vi "ALTS-2015 Check Robot Requests.vi"(8 "error in (no error)":errorcluster, 10 "Data Cluster in":T1, 11 "Cases to go in":string) -> (0 "error out":errorcluster, 2 "Data Cluster out":T1, 3 "Cases to go out":string)   [LabVIEW 2013]
uses:
  Controls/ALTS-2015 Data Cluster.ctl
  Controls/ALTS-2015 Station Cluster.ctl
  Controls/ALTS-2015 INI Configuration Cluster.ctl
  Controls/ALTS-2015 Unload Task Data.ctl
  OPC Engine/Controls/ALTS-2015 OPC Read Registers.ctl
  OPC Engine/Controls/ALTS-2015 OPC Read Global Options.ctl
  Controls/ALTS-2015 Auto Main Screen States.ctl
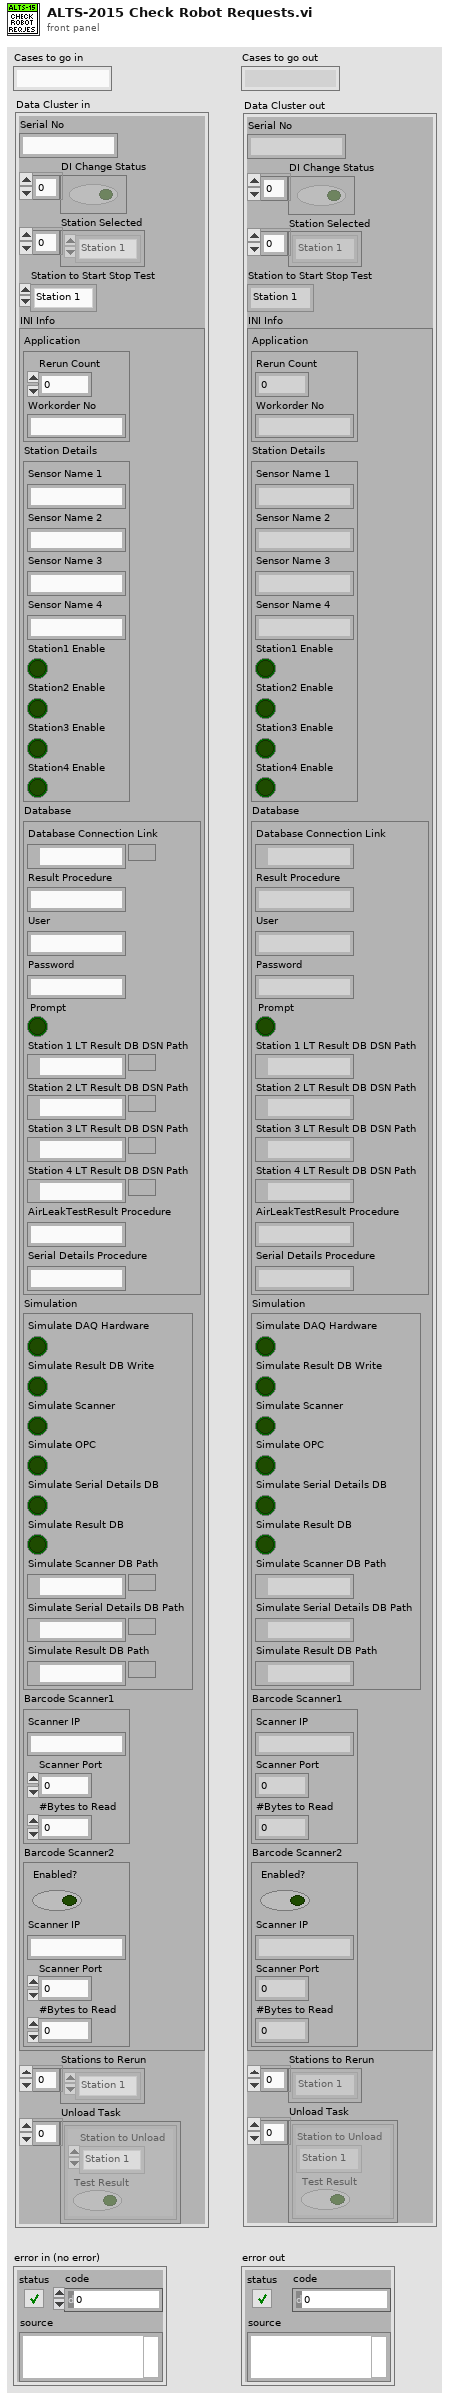
[diagram p1: front panel]
types:
  T1 = typedef "ALTS-2015 Data Cluster.ctl" = cluster{"Serial No":string, "DI Change Status":bool[], "Station Selected":T2[], "Station to Start Stop Test":T2, "INI Info":T3, "Stations to Rerun":T2[], "Unload Task":T4[]}
  T2 = typedef "ALTS-2015 Station Cluster.ctl" = enum16{"Station 1", "Station 2", "Station 3", "Station 4"}
  T3 = typedef "ALTS-2015 INI Configuration Cluster.ctl" = cluster{"Application":cluster{"Rerun Count":i32, "Workorder No":string}, "Station Details":cluster{"Sensor Name 1":string, "Sensor Name 2":string, "Sensor Name 3":string, "Sensor Name 4":string, "Station1 Enable":bool, "Station2 Enable":bool, "Station3 Enable":bool, "Station4 Enable":bool}, "Database":cluster{"Database Connection Link":path, "Result Procedure":string, "User":string, "Password":string, "Prompt":bool, "Station 1 LT Result DB DSN Path":path, "Station 2 LT Result DB DSN Path":path, "Station 3 LT Result DB DSN Path":path, "Station 4 LT Result DB DSN Path":path, "AirLeakTestResult Procedure":string, "Serial Details Procedure":string}, "Simulation":cluster{"Simulate DAQ Hardware":bool, "Simulate Result DB Write":bool, "Simulate Scanner":bool, "Simulate OPC":bool, "Simulate Serial Details DB":bool, "Simulate Result DB":bool, "Simulate Scanner DB Path":path, "Simulate Serial Details DB Path":path, "Simulate Result DB Path":path}, "Barcode Scanner1":cluster{"Scanner IP":string, "Scanner Port":u16, "#Bytes to Read":i32}, "Barcode Scanner2":cluster{"Enabled?":bool, "Scanner IP":string, "Scanner Port":u16, "#Bytes to Read":i32}}
  T4 = typedef "ALTS-2015 Unload Task Data.ctl" = cluster{"Station to Unload":T2, "Test Result":bool}
  T5 = typedef "ALTS-2015 OPC Read Global Options.ctl" = enum16{"Init", "Write Value", "Write Array", "Read Value", "Read Array", "Read All"}
  T6 = typedef "ALTS-2015 OPC Read Registers.ctl" = enum16{"Robot_Available", "Start_Test", "Stop_Test", "Scan_Trigger", "Station_No_Start_Stop_Test"}
  T7 = typedef "ALTS-2015 Auto Main Screen States.ctl" = enum16{">Initialize", ">Poll", ">Error", ">Exit", ">Authentication", ">Initial FP Update", ">Check Robot Requests", ">Scan Serial No", "<-------DI /OPC Actions------->", ">Check DI Status", ">Start the Test", ">Restore station after Stop", ">Stop the Test", ">UUT Clamped", ">UUT Unclamped", ">Read Test Data Result - Pass", ">Read Test Data Result - Fail", ">Update Rerun on Fail", ">Update Station Info", "<--------Enqueue Robot Task-------->", ">Enqueue New Serial Task", ">Enqueue Invalid Serial Task", ">Enqueue Rerun Task", ">Enqueu Unload Task"}
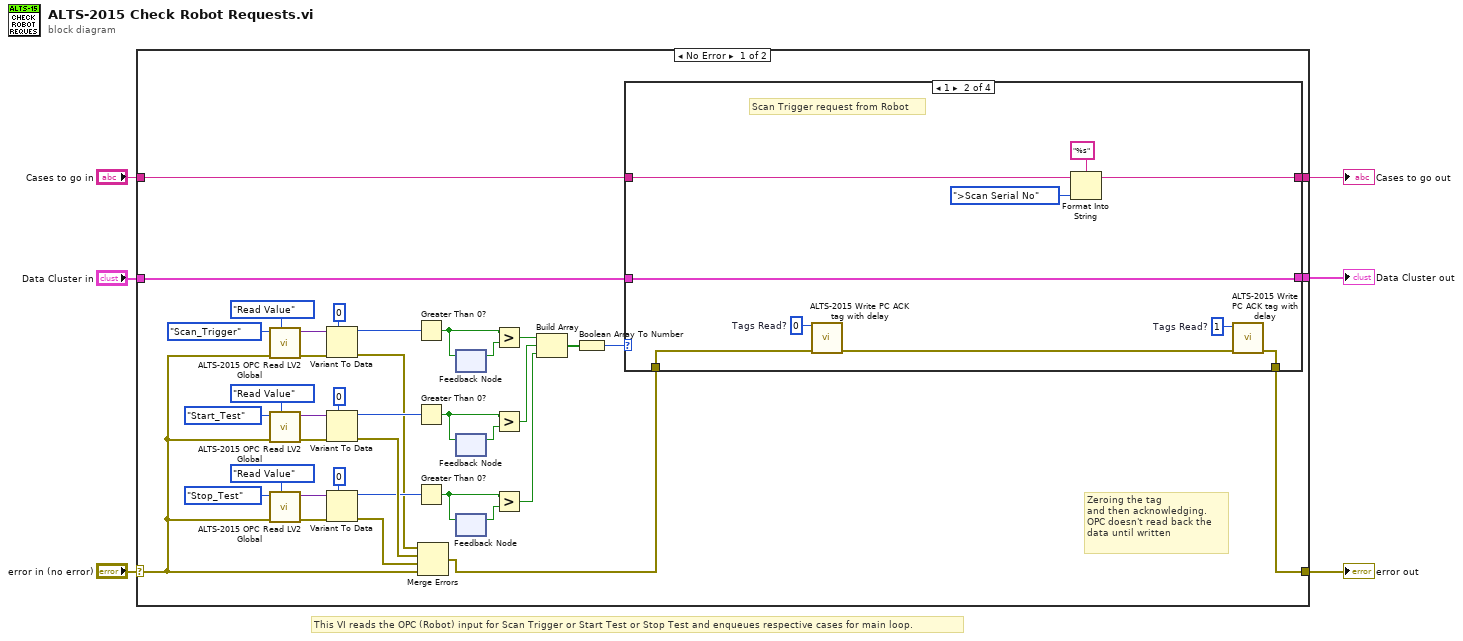
[diagram p0: block diagram]
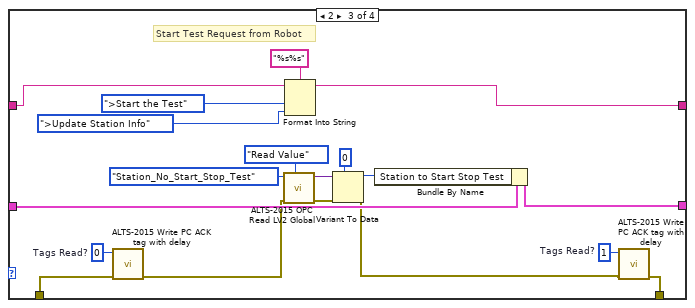
[diagram p3: hidden frame]
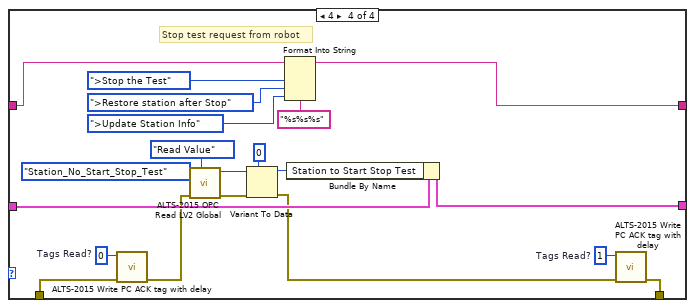
[diagram p4: hidden frame]
diagram:
  # "This VI reads the OPC (Robot) input for Scan Trigger or Start Test or Stop Test and enqueues respective cases for main loop."
  n1 = case shown="No Error" "error in (no error)" {
    selector: "error in (no error)" -> [w11 w100]
    tunnel: [w8 w100] -> w6
    tunnel: [w43 w98] -> w5
    tunnel: "Data Cluster in" -> [w42 w98]
    tunnel: [w41 w99] -> w3
    tunnel: "Cases to go in" -> [w40 w99]
    frame No Error {
      # "Zeroing the tag\nand then acknowledging.\nOPC doesn't read back the\ndata until written"
      n2 = call "ALTS-2015 OPC Read LV2 Global.vi"("Options"=ALTS-2015_OPC_Read_Global_Options."Read Value", "error in (no error)"=w11, "OPC Read Register"=ALTS-2015_OPC_Read_Registers."Scan_Trigger") -> ("error out"=w15:errorcluster, "OPC Read Reigter Value"=w16:variant)  [unwired: 6 in, 1 out]
      n3 = call "ALTS-2015 OPC Read LV2 Global.vi"("Options"=ALTS-2015_OPC_Read_Global_Options."Read Value", "error in (no error)"=w11, "OPC Read Register"=ALTS-2015_OPC_Read_Registers."Start_Test") -> ("error out"=w21:errorcluster, "OPC Read Reigter Value"=w20:variant)  [unwired: 6 in, 1 out]
      n4 = call "ALTS-2015 OPC Read LV2 Global.vi"("Options"=ALTS-2015_OPC_Read_Global_Options."Read Value", "error in (no error)"=w11, "OPC Read Register"=ALTS-2015_OPC_Read_Registers."Stop_Test") -> ("error out"=w37:errorcluster, "OPC Read Reigter Value"=w38:variant)  [unwired: 6 in, 1 out]
      n5 = Variant To Data(error in=w15, type=0, Variant=w16) -> (data=w17:i32, error out=w7:errorcluster)
      n6 = Variant To Data(error in=w21, type=0, Variant=w20) -> (data=w27:i32, error out=w44:errorcluster)
      n7 = Variant To Data(error in=w37, type=0, Variant=w38) -> (data=w31:i32, error out=w45:errorcluster)
      n8 = Greater Than 0?(x=w17) -> (x > 0?=w18:bool)
      n9 = Greater Than 0?(x=w27) -> (x > 0?=w26:bool)
      n10 = Greater Than 0?(x=w31) -> (x > 0?=w32:bool)
      n11 = Merge Errors(w7, w44, w45, w11) -> (w9:errorcluster)
      n12 = feedback #1() -> (w19:bool)  [unwired: 1 in]
      n13 = feedback-in #1(w18) -> ()
      n14 = feedback #2() -> (w25:bool)  [unwired: 1 in]
      n15 = feedback-in #2(w26) -> ()
      n16 = feedback #3() -> (w33:bool)  [unwired: 1 in]
      n17 = feedback-in #3(w32) -> ()
      n18 = Greater?(x=w18, y=w19) -> (0:w29:bool)
      n19 = Greater?(x=w26, y=w25) -> (0:w28:bool)
      n20 = Greater?(x=w32, y=w33) -> (0:w39:bool)
      n21 = Build Array(w29, w28, w39) -> (w30:bool[])
      n22 = Boolean Array To Number(Boolean array=w30) -> (number=w10:u32)
      n23 = case shown="1" w10 {
        tunnel: [w48 w57 w76 w96] -> w41
        tunnel: w40 -> [w48 w56 w75 w95]
        tunnel: w42 -> [w47 w54 w66 w87]
        tunnel: [w47 w54 w65 w86] -> w43
        tunnel: w9 -> [w46 w52 w64 w83]
        tunnel: [w46 w53 w61 w81] -> w8
        frame 0, Default {
          # "No Request from Robot"
        }
        frame 1 {
          w49 = 0  # Tags Read?
          w51 = 1  # Tags Read?
          # "Scan Trigger request from Robot"
          n24 = call "ALTS-2015 Write PC ACK tag with delay.vi"("error in (no error)"=w52, "Tags Read?"=w49) -> ("error out"=w50:errorcluster)  [unwired: 9 in]
          n25 = Format Into String(format string="%s", initial string=w56, ALTS-2015_Auto_Main_Screen_States.">Scan Serial No") -> (resulting string=w57:string)  [unwired: 1 in, 1 out]
          n26 = call "ALTS-2015 Write PC ACK tag with delay.vi"("error in (no error)"=w50, "Tags Read?"=w51) -> ("error out"=w53:errorcluster)  [unwired: 9 in]
        }
        frame 2 {
          w59 = 0  # Tags Read?
          w63 = 1  # Tags Read?
          # "Start Test Request from Robot"
          n27 = call "ALTS-2015 Write PC ACK tag with delay.vi"("error in (no error)"=w64, "Tags Read?"=w59) -> ("error out"=w60:errorcluster)  [unwired: 9 in]
          n28 = call "ALTS-2015 OPC Read LV2 Global.vi"("Options"=ALTS-2015_OPC_Read_Global_Options."Read Value", "error in (no error)"=w60, "OPC Read Register"=ALTS-2015_OPC_Read_Registers."Station_No_Start_Stop_Test") -> ("error out"=w72:errorcluster, "OPC Read Reigter Value"=w73:variant)  [unwired: 6 in, 1 out]
          n29 = Format Into String(format string="%s%s", initial string=w75, ALTS-2015_Auto_Main_Screen_States.">Start the Test", ALTS-2015_Auto_Main_Screen_States.">Update Station Info") -> (resulting string=w76:string)  [unwired: 1 in, 1 out]
          n30 = Variant To Data(error in=w72, type=0, Variant=w73) -> (data=w68:i32, error out=w62:errorcluster)
          n31 = Bundle By Name(cluster=w66, "Station to Start Stop Test"=w68) -> (w65:T1)
          n32 = call "ALTS-2015 Write PC ACK tag with delay.vi"("error in (no error)"=w62, "Tags Read?"=w63) -> ("error out"=w61:errorcluster)  [unwired: 9 in]
        }
        frame 4 {
          w78 = 0  # Tags Read?
          w80 = 1  # Tags Read?
          # "Stop test request from robot"
          n33 = call "ALTS-2015 Write PC ACK tag with delay.vi"("error in (no error)"=w83, "Tags Read?"=w78) -> ("error out"=w79:errorcluster)  [unwired: 9 in]
          n34 = call "ALTS-2015 OPC Read LV2 Global.vi"("Options"=ALTS-2015_OPC_Read_Global_Options."Read Value", "error in (no error)"=w79, "OPC Read Register"=ALTS-2015_OPC_Read_Registers."Station_No_Start_Stop_Test") -> ("error out"=w92:errorcluster, "OPC Read Reigter Value"=w93:variant)  [unwired: 6 in, 1 out]
          n35 = Variant To Data(error in=w92, type=0, Variant=w93) -> (data=w88:i32, error out=w82:errorcluster)
          n36 = Format Into String(format string="%s%s%s", initial string=w95, ALTS-2015_Auto_Main_Screen_States.">Stop the Test", ALTS-2015_Auto_Main_Screen_States.">Restore station after Stop", ALTS-2015_Auto_Main_Screen_States.">Update Station Info") -> (resulting string=w96:string)  [unwired: 1 in, 1 out]
          n37 = Bundle By Name(cluster=w87, "Station to Start Stop Test"=w88) -> (w86:T1)
          n38 = call "ALTS-2015 Write PC ACK tag with delay.vi"("error in (no error)"=w82, "Tags Read?"=w80) -> ("error out"=w81:errorcluster)  [unwired: 9 in]
        }
      }
    }
    frame Error {
    }
  }
  "error out" <- w6
  "Data Cluster out" <- w5
  "Cases to go out" <- w3
